vi "subTrimWaveform.vi"(0 "input waveform":cdb[][](array[numeric]) format="%#_6p", 5 "magnitude threshold (of peak)":dbl=0.05, 7 "hysteresis":i32=10, 11 "error in (no error)":errorcluster) -> (4 "output waveform":cdb[][](array[numeric]) format="%#_6p", 15 "error out":errorcluster)   [LabVIEW 2011]
uses:
  packetDetectionState.ctl
panel:
  out "max value":i32
  out "min value":i32
  in  "detection state":T1
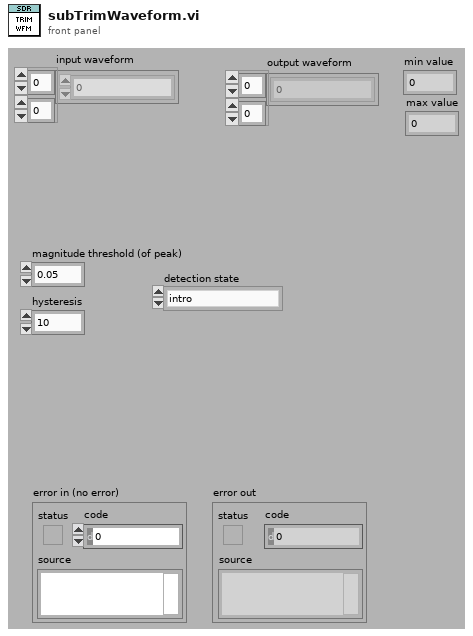
[diagram p1: front panel]
types:
  T1 = typedef "packetDetectionState.ctl" = enum16{"intro", "pre-packet", "test packet entry", "packet", "test packet exit", "post-packet"}
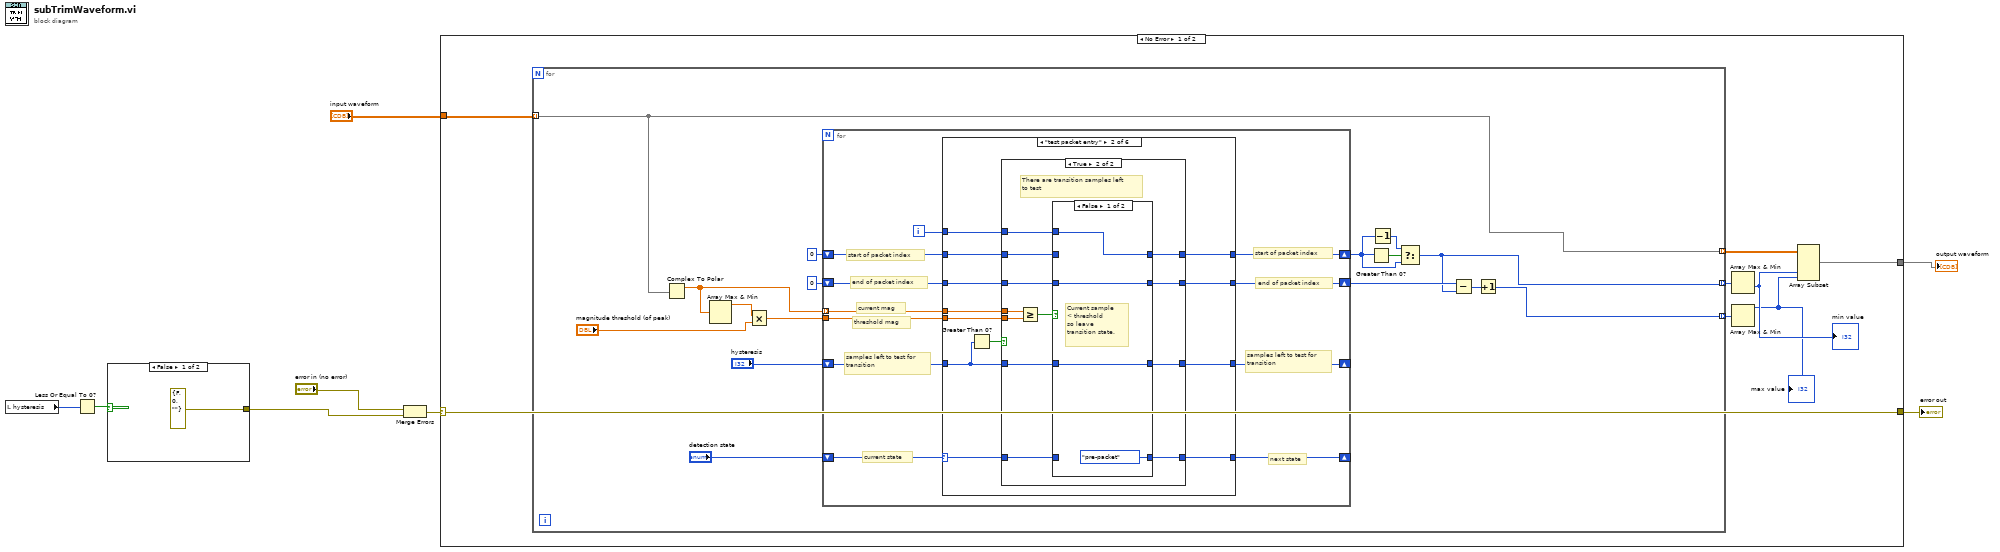
[diagram p0: block diagram]
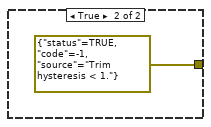
[diagram p2: hidden frame]
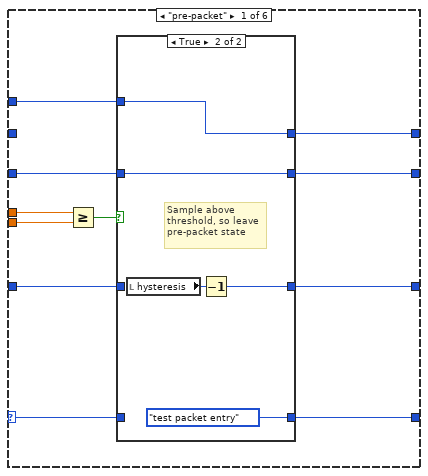
[diagram p3: hidden frame]
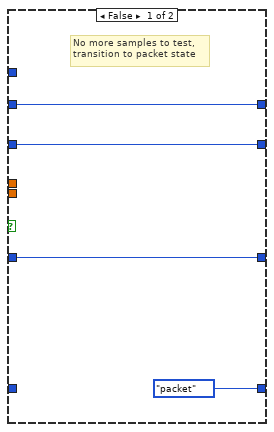
[diagram p5: hidden frame]
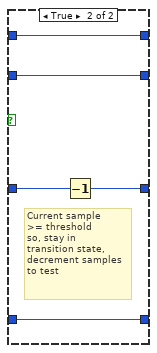
[diagram p6: hidden frame]
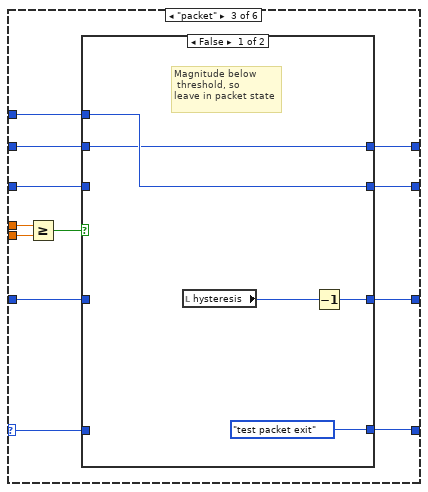
[diagram p7: hidden frame]
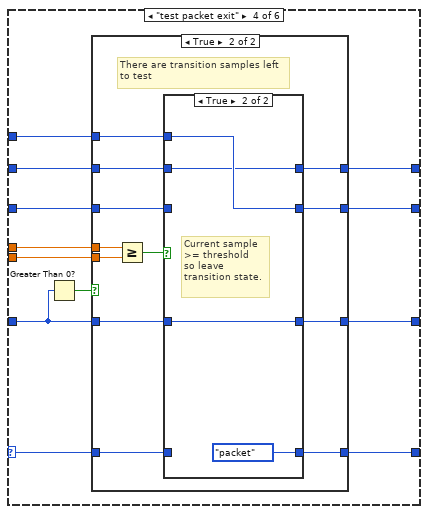
[diagram p9: hidden frame]
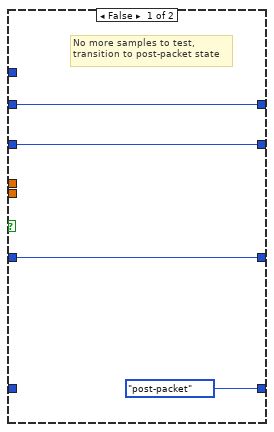
[diagram p10: hidden frame]
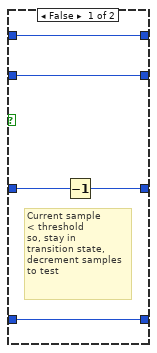
[diagram p11: hidden frame]
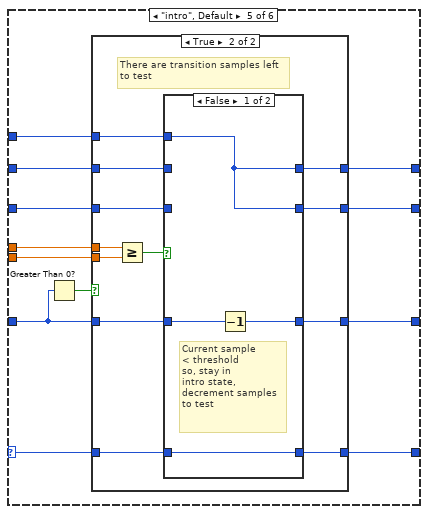
[diagram p12: hidden frame]
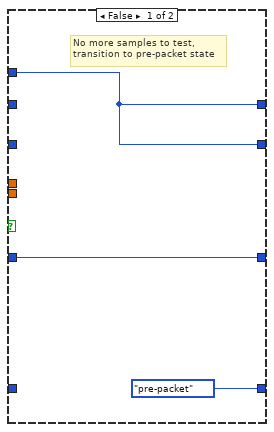
[diagram p13: hidden frame]
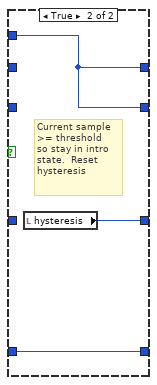
[diagram p14: hidden frame]
diagram:
  n1 = local read "hysteresis"() -> (w6:i32)
  n2 = Less Or Equal To 0?(x=w6) -> (x <= 0?=w7:bool)
  n3 = case shown="False" w7 {
    tunnel: [errorcluster {"status"=FALSE, "code"=0, "source"=""} ("error in (no error)") errorcluster {"status"=TRUE, "code"=-1, "source"="Trim hysteresis < 1."} ("error in (no error)")] -> w3
    frame False {
    }
    frame True {
    }
  }
  n4 = Merge Errors("error in (no error)", w3) -> (w4:errorcluster)
  n5 = case shown="No Error" w4 {
    selector: w4 -> [w18 w199]
    tunnel: [w18 w199] -> w8
    tunnel: [w12 _] -> w2
    tunnel: "input waveform" -> [w11 _]
    frame No Error {
      n6 = for {
        tunnel: w11 -> [w19] mode=indexing
        tunnel: [w19] -> w17 mode=indexing
        tunnel: [w21] -> w15 mode=indexing
        tunnel: [w20] -> w16 mode=indexing
        n7 = Complex To Polar(r * e^(i*theta)=w19) -> (r=w25:dbl[])  [unwired: 1 out]
        n8 = Array Max & Min(array=w25) -> (max value=w24:dbl)  [unwired: 3 out]
        n9 = Multiply(x=w24, y="magnitude threshold (of peak)") -> (x*y=w22:dbl)
        n10 = for {
          tunnel: w25 -> [w44] mode=indexing
          shift-right: [w42] -> _
          shift-left: "detection state" -> [w45]
          tunnel: w22 -> [w43]
          shift-right: [w41] -> _
          shift-left: "hysteresis" -> [w40]
          shift-right: [w38] -> w28
          shift-left: 0 -> [w37]
          shift-right: [w36] -> w32
          shift-left: 0 -> [w35]
          i -> [w39]
          # "current state"
          # "samples left to test for\ntransition"
          # "threshold mag"
          # "current mag"
          # "end of packet index"
          # "start of packet index"
          # "end of packet index"
          # "start of packet index"
          # "next state"
          # "samples left to test for\ntransition"
          n11 = case shown="\"test packet entry\"" w45 {
            selector: w45 -> [w50 w74 w107 w132 w169 w195]
            tunnel: w44 -> [w56 w76 w113 w134 w171 _]
            tunnel: w43 -> [w55 w75 w114 w133 w170 _]
            tunnel: [w53 w73 w106 w131 w168 w195] -> w42
            tunnel: [w52 w68 w108 w126 w163 w196] -> w41
            tunnel: w40 -> [w51 w69 w109 w127 w164 w196]
            tunnel: w39 -> [w49 w70 w105 w128 w165 _]
            tunnel: [w48 w71 w110 w129 w166 w198] -> w38
            tunnel: w37 -> [_ w72 w111 w130 w167 w198]
            tunnel: [w46 w66 w104 w124 w161 w197] -> w36
            tunnel: w35 -> [w47 w67 w103 w125 w162 w197]
            frame "pre-packet" {
              n12 = Greater Or Equal?(x=w56, y=w55) -> (x >= y?=w54:bool)
              n13 = case shown="True" w54 {
                tunnel: [w59 packetDetectionState."test packet entry" ("detection state")] -> w53
                tunnel: [w60 w65] -> w52
                tunnel: w51 -> [w60 _]
                tunnel: w50 -> [w59 _]
                tunnel: w49 -> [w58 w64]
                tunnel: [w58 w64] -> w48
                tunnel: [w57 w63] -> w46
                tunnel: w47 -> [w57 w63]
                frame False {
                  # "Sample not\nabove threshold\nso stay in pre-packet\nstate."
                }
                frame True {
                  # "Sample above \nthreshold, so leave\npre-packet state"
                  n14 = local read "hysteresis"() -> (w61:i32)
                  n15 = Decrement(x=w61) -> (x-1=w65:i32)
                }
              }
            }
            frame "test packet entry" {
              n16 = Greater Than 0?(x=w69) -> (x > 0?=w77:bool)
              n17 = case shown="True" w77 {
                tunnel: w76 -> [_ w93]
                tunnel: w75 -> [_ w92]
                tunnel: [packetDetectionState."packet" ("detection state") w89] -> w73
                tunnel: w74 -> [_ w90]
                tunnel: w72 -> [w81 w88]
                tunnel: [w81 w87] -> w71
                tunnel: w70 -> [_ w86]
                tunnel: [w80 w84] -> w68
                tunnel: w69 -> [w80 w85]
                tunnel: w67 -> [w79 w83]
                tunnel: [w79 w82] -> w66
                frame False {
                  # "No more samples to test, \ntransition to packet state"
                }
                frame True {
                  # "There are transition samples left\nto test"
                  n18 = Greater Or Equal?(x=w93, y=w92) -> (x >= y?=w91:bool)
                  n19 = case shown="False" w91 {
                    tunnel: [packetDetectionState."pre-packet" ("detection state") w102] -> w89
                    tunnel: w90 -> [_ w102]
                    tunnel: w88 -> [_ w101]
                    tunnel: [w97 w101] -> w87
                    tunnel: w86 -> [w97 _]
                    tunnel: [w96 w99] -> w84
                    tunnel: w85 -> [w96 w100]
                    tunnel: [w95 w98] -> w82
                    tunnel: w83 -> [w95 w98]
                    frame False {
                      # "Current sample \n< threshold\nso leave \ntransition state."
                    }
                    frame True {
                      # "Current sample \n>= threshold\nso, stay in \ntransition state, \ndecrement samples\nto test"
                      n20 = Decrement(x=w100) -> (x-1=w99:i32)
                    }
                  }
                }
              }
            }
            frame "packet" {
              n21 = Greater Or Equal?(x=w113, y=w114) -> (x >= y?=w112:bool)
              n22 = case shown="False" w112 {
                tunnel: [w116 w123] -> w110
                tunnel: w111 -> [w116 w123]
                tunnel: [w118 w122] -> w108
                tunnel: w109 -> [_ w122]
                tunnel: [packetDetectionState."test packet exit" ("detection state") w121] -> w106
                tunnel: w107 -> [_ w121]
                tunnel: [w119 w120] -> w104
                tunnel: w105 -> [w119 w120]
                tunnel: w103 -> [_ _]
                frame False {
                  # "Magnitude below\n threshold, so \nleave in packet state"
                  n23 = local read "hysteresis"() -> (w117:i32)
                  n24 = Decrement(x=w117) -> (x-1=w118:i32)
                }
                frame True {
                  # "Magnitude still \nabove threshold, so \nstay in packet state"
                }
              }
            }
            frame "test packet exit" {
              n25 = Greater Than 0?(x=w127) -> (x > 0?=w135:bool)
              n26 = case shown="True" w135 {
                tunnel: w134 -> [_ w151]
                tunnel: w133 -> [_ w150]
                tunnel: [packetDetectionState."post-packet" ("detection state") w147] -> w131
                tunnel: w132 -> [_ w148]
                tunnel: w130 -> [w139 w146]
                tunnel: [w139 w145] -> w129
                tunnel: w128 -> [_ w144]
                tunnel: [w138 w142] -> w126
                tunnel: w127 -> [w138 w143]
                tunnel: w125 -> [w137 w141]
                tunnel: [w137 w140] -> w124
                frame False {
                  # "No more samples to test, \ntransition to post-packet state"
                }
                frame True {
                  # "There are transition samples left\nto test"
                  n27 = Greater Or Equal?(x=w151, y=w150) -> (x >= y?=w149:bool)
                  n28 = case shown="True" w149 {
                    tunnel: [w156 packetDetectionState."packet" ("detection state")] -> w147
                    tunnel: w148 -> [w156 _]
                    tunnel: w146 -> [w155 w158]
                    tunnel: [w155 w158] -> w145
                    tunnel: w144 -> [_ w159]
                    tunnel: [w153 w160] -> w142
                    tunnel: w143 -> [w154 w160]
                    tunnel: [w152 w159] -> w140
                    tunnel: w141 -> [w152 _]
                    frame False {
                      # "Current sample \n< threshold\nso, stay in \ntransition state, \ndecrement samples\nto test"
                      n29 = Decrement(x=w154) -> (x-1=w153:i32)
                    }
                    frame True {
                      # "Current sample \n>= threshold\nso leave \ntransition state."
                    }
                  }
                }
              }
            }
            frame "intro", Default {
              n30 = Greater Than 0?(x=w164) -> (x > 0?=w172:bool)
              n31 = case shown="True" w172 {
                tunnel: w171 -> [_ w187]
                tunnel: w170 -> [_ w186]
                tunnel: [packetDetectionState."pre-packet" ("detection state") w183] -> w168
                tunnel: w169 -> [_ w184]
                tunnel: w167 -> [_ w182]
                tunnel: [w173 w181] -> w166
                tunnel: w165 -> [w173 w180]
                tunnel: [w175 w178] -> w163
                tunnel: w164 -> [w175 w179]
                tunnel: w162 -> [_ w177]
                tunnel: [w173 w176] -> w161
                frame False {
                  # "No more samples to test, \ntransition to pre-packet state"
                }
                frame True {
                  # "There are transition samples left\nto test"
                  n32 = Greater Or Equal?(x=w187, y=w186) -> (x >= y?=w185:bool)
                  n33 = case shown="False" w185 {
                    tunnel: [w191 w192] -> w183
                    tunnel: w184 -> [w191 w192]
                    tunnel: w182 -> [_ _]
                    tunnel: [w188 w194] -> w181
                    tunnel: w180 -> [w188 w194]
                    tunnel: [w189 w193] -> w178
                    tunnel: w179 -> [w190 _]
                    tunnel: [w188 w194] -> w176
                    tunnel: w177 -> [_ _]
                    frame False {
                      # "Current sample \n< threshold\nso, stay in \nintro state, \ndecrement samples\nto test"
                      n34 = Decrement(x=w190) -> (x-1=w189:i32)
                    }
                    frame True {
                      # "Current sample \n>= threshold\nso stay in intro\nstate.  Reset \nhysteresis"
                      n35 = local read "hysteresis"() -> (w193:i32)
                    }
                  }
                }
              }
            }
            frame "post-packet" {
            }
          }
        }
        n36 = Greater Than 0?(x=w28) -> (x > 0?=w30:bool)
        n37 = Decrement(x=w28) -> (x-1=w29:i32)
        n38 = Select(t=w29, s=w30, f=w28) -> (s? t:f=w21:i32)
        n39 = Subtract(x=w32, y=w21) -> (x-y=w31:i32)
        n40 = Increment(x=w31) -> (x+1=w20:i32)
      }
      n41 = Array Max & Min(array=w15) -> (min value=w14:i32)  [unwired: 3 out]
      "min value" <- w14
      n42 = Array Max & Min(array=w16) -> (max value=w13:i32)  [unwired: 3 out]
      "max value" <- w13
      n43 = Array Subset(array=w17, index (col)=w14, length (col)=w13) -> (w12:cdb[][])  [unwired: 2 in]
    }
    frame Error {
    }
  }
  "error out" <- w8
  "output waveform" <- w2
